vi "Create.vi"(7 "fifo options":T1, 8 "error in (no error)":errorcluster, 11 "fifo/queue depths (10)":u32=10) -> (0 "error out":errorcluster, 3 "Logging Interface out":refnum<class "Logging Interface.lvclass">)   [LabVIEW 2021, in "DSF Core.lvlib" / "Logging Interface.lvclass"]
uses:
  Logging Interface.lvclass
  C:/dev/git/custom-devices/niveristand-data-sharing-framework-custom-device/Source/Core/Classes/Interface/Interface.lvclass
  Typedefs/DSF FIFO Options.ctl
  Response Data.ctl
  Response.ctl
  Parameters.ctl
  Command Data.ctl
  Command.ctl
  FIFO Descriptors.ctl
  FIFO Descriptor.ctl
  Interface.lvclass/Interface.ctl
  Create RT FIFO.vi
  Interface.lvclass
  Framework/Framework.lvclass
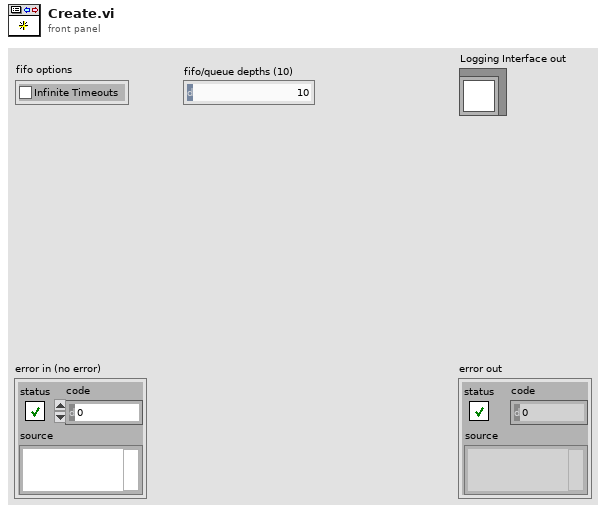
[diagram p1: front panel]
types:
  T1 = typedef "DSF Core.lvlib/Framework.lvclass/DSF FIFO Options.ctl" = cluster{"Infinite Timeouts":bool}
  T2 = typedef "DSF Core.lvlib/Logging Interface.lvclass/Response Data.ctl" = cluster{"Response":T3, "Parameters":T4}
  T3 = typedef "DSF Core.lvlib/Logging Interface.lvclass/Response.ctl" = enum8{"General Ack", "Error", "Shutting Down"}
  T4 = typedef "DSF Core.lvlib/Logging Interface.lvclass/Parameters.ctl" = cluster{"arg1":u64, "arg2":u64}
  T5 = typedef "DSF Core.lvlib/Logging Interface.lvclass/Command Data.ctl" = cluster{"Command":T6, "Parameters":T4}
  T6 = typedef "DSF Core.lvlib/Logging Interface.lvclass/Command.ctl" = enum8{"Idle", "Start", "Log Framework State", "Log Plugin State", "Log Dispatcher State", "Shutdown"}
  T7 = typedef "DSF Core.lvlib/Interface.lvclass/FIFO Descriptors.ctl" = cluster{"command fifo":T8, "response fifo":T8, "error fifo":T8}
  T8 = typedef "DSF Core.lvlib/Interface.lvclass/FIFO Descriptor.ctl" = cluster{"fifo depth":u32, "element size":u32}
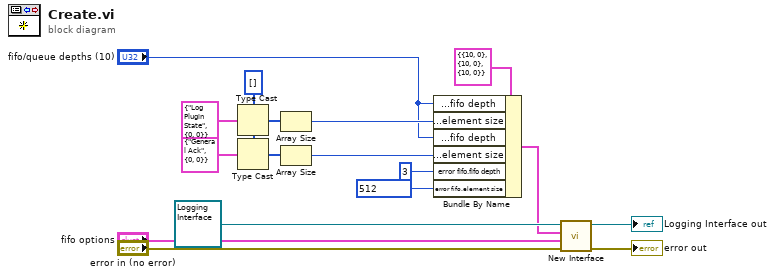
[diagram p0: block diagram]
diagram:
  w5 = u8[] [] ("element")
  n1 = Type Cast(type=w5, x=T5 {"Command"=enum."Log Plugin State", "Parameters"={"arg1"=0, "arg2"=0}} ("Logging Command")) -> (*(type *) &x=w11:u8[])
  n2 = Type Cast(type=w5, x=T2 {"Response"=enum."General Ack", "Parameters"={"arg1"=0, "arg2"=0}} ("Dispatcher Response")) -> (*(type *) &x=w9:u8[])
  n3 = Array Size(array=w11) -> (size(s)=w10:i32)
  n4 = Array Size(array=w9) -> (size(s)=w7:i32)
  n5 = Bundle By Name(cluster=T7 {"command fifo"={"fifo depth"=10, "element size"=0}, "response fifo"={"fifo depth"=10, "element size"=0}, "error fifo"={"fifo depth"=10, "element size"=0}} ("fifo descriptors"), "command fifo.fifo depth"="fifo/queue depths (10)", "command fifo.element size"=w10, "response fifo.fifo depth"="fifo/queue depths (10)", "response fifo.element size"=w7, "error fifo.fifo depth"=u32 3, "error fifo.element size"=u32 512 ("element size")) -> (w1:T7)
  n6 = call "New Interface.vi"("error in (no error)"="error in (no error)", "fifo options"="fifo options", "fifo descriptors"=w1, "Interface type"=refnum<class "Logging Interface.lvclass"> refnum ("Logging Interface in")) -> ("error out"=→"error out":errorcluster, "Interface"=→"Logging Interface out":refnum<class "Logging Interface.lvclass">)  [unwired: 6 in]
